vi "ParkFXP_src.vi"(0 "alpha":fxp<+/-,32,4> format="%#_32g", 5 "beta":fxp<+/-,32,4> format="%#_32g", 7 "theta":fxp<+/-,16,1>) -> (4 "direct":fxp<+/-,32,4>, 6 "quadrature":fxp<+/-,32,4>)   [LabVIEW 2016]
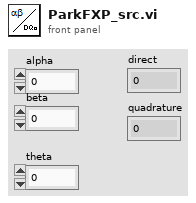
[diagram p1: front panel]
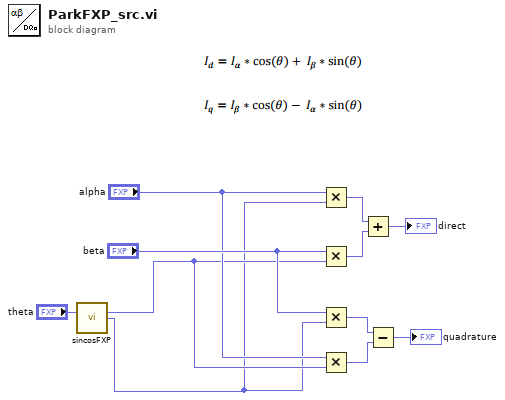
[diagram p0: block diagram]
diagram:
  n1 = call "sincosFXP.vi"("x"="theta") -> ("sinx"=w3:fxp<+/-,16,2>, "cosx"=w2:fxp<+/-,16,2>)  [unwired: 13 in]
  n2 = Multiply(x="alpha", y=w2) -> (x*y=w9:fxp<+/-,32,4>)
  n3 = Multiply(x="beta", y=w3) -> (x*y=w8:fxp<+/-,32,4>)
  n4 = Multiply(x="beta", y=w2) -> (x*y=w7:fxp<+/-,32,4>)
  n5 = Multiply(x="alpha", y=w3) -> (x*y=w6:fxp<+/-,32,4>)
  n6 = Add(x=w9, y=w8) -> (x+y=→"direct":fxp<+/-,32,4>)
  n7 = Subtract(x=w7, y=w6) -> (x-y=→"quadrature":fxp<+/-,32,4>)
